vi "3_2_(1).vi"() -> ()   [LabVIEW 2010]
uses:
  Control 1.ctl
  Global 1.vi
panel:
  in  "Зчитати дані":bool
  out "Таблиця 1 - Вхідні дані":string[][](table)
  out "Таблиця 2 - Сортування":string[][](table)
  in  "4":bool
  in  "3":bool
  in  "2":bool
  in  "1":bool
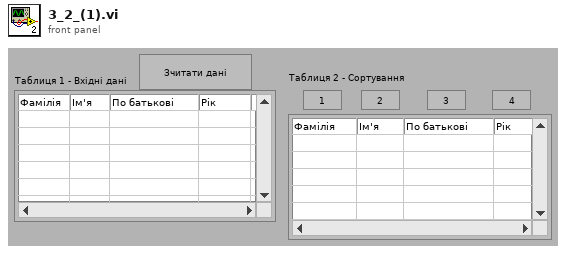
[diagram p1: front panel]
types:
  T1 = typedef "Control 1.ctl" = enum16{"Зчитати", "Стоп", "1", "2", "3", "4"}
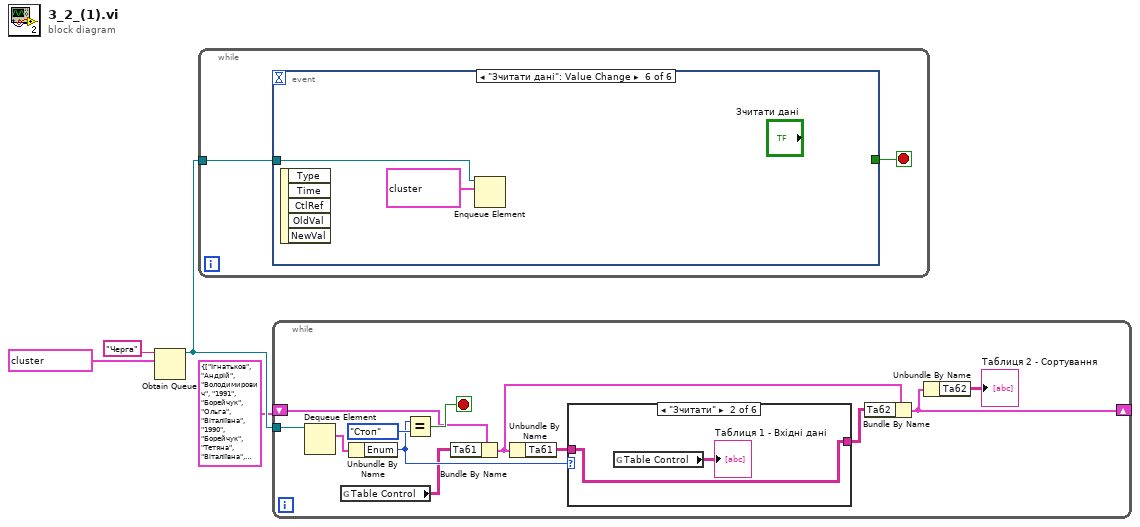
[diagram p0: block diagram]
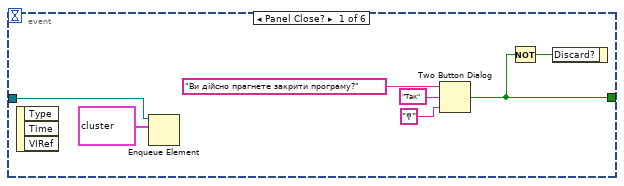
[diagram p2: hidden frame]
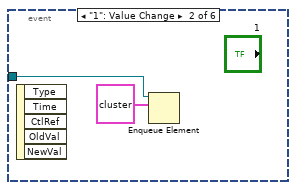
[diagram p3: hidden frame]
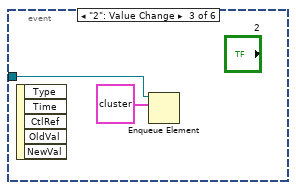
[diagram p4: hidden frame]
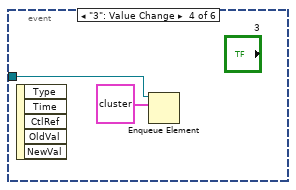
[diagram p5: hidden frame]
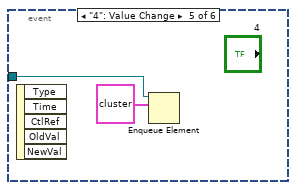
[diagram p6: hidden frame]
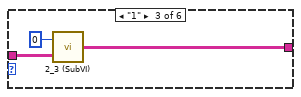
[diagram p8: hidden frame]
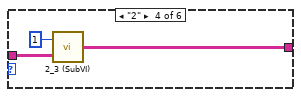
[diagram p9: hidden frame]
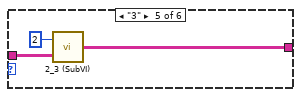
[diagram p10: hidden frame]
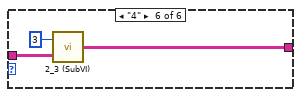
[diagram p11: hidden frame]
diagram:
  n1 = Obtain Queue(name (unnamed)="Черга", element data type=cluster{"variant":variant, "Enum":T1} {"variant"=variant, "Enum"=enum."Стоп"}) -> (queue out=w2:refnum<queue>)  [unwired: 3 in, 2 out]
  n2 = while {
    tunnel: w2 -> [w5]
    stop <- w6 stop-if-true
    n3 = event shown="[5] \"Зчитати дані\": Value Change" {
      selector: _ -> [_ _ _ _ _ _]
      dyn-events: _ -> [_ _ _ _ _ _]
      timeout: _ -> [_ _ _ _ _ _]
      tunnel: [w9 _ _ _ _ _] -> w6
      tunnel: w5 -> [w8 w14 w16 w18 w20 w22]
      event Panel Close? {
        n4 = event-data() -> ()  [unwired: 1 in, 3 out]
        n5 = Enqueue Element(queue=w8, element=cluster{"variant":variant, "Enum":T1} {"variant"=variant, "Enum"=enum."Стоп"}) -> ()  [unwired: 2 in, 3 out]
        n6 = Two Button Dialog(message="Ви дійсно прагнете закрити програму?", 1:"ͳ" ("F button name (\"Cancel\")"), 2:"Так" ("T button name (\"OK\")")) -> (T button?=w9:bool)
        n7 = Not(x=w9) -> (.not. x?=w10:bool)
        n8 = event-data("Discard?"=w10) -> ()  [unwired: 1 in, 1 out]
      }
      event "1": Value Change {
        n9 = event-data() -> ()  [unwired: 1 in, 5 out]
        n10 = Enqueue Element(queue=w14, element=cluster{"variant":variant, "Enum":T1} {"variant"=variant, "Enum"=enum."1"}) -> ()  [unwired: 2 in, 3 out]
      }
      event "2": Value Change {
        n11 = event-data() -> ()  [unwired: 1 in, 5 out]
        n12 = Enqueue Element(queue=w16, element=cluster{"variant":variant, "Enum":T1} {"variant"=variant, "Enum"=enum."2"}) -> ()  [unwired: 2 in, 3 out]
      }
      event "3": Value Change {
        n13 = event-data() -> ()  [unwired: 1 in, 5 out]
        n14 = Enqueue Element(queue=w18, element=cluster{"variant":variant, "Enum":T1} {"variant"=variant, "Enum"=enum."3"}) -> ()  [unwired: 2 in, 3 out]
      }
      event "4": Value Change {
        n15 = event-data() -> ()  [unwired: 1 in, 5 out]
        n16 = Enqueue Element(queue=w20, element=cluster{"variant":variant, "Enum":T1} {"variant"=variant, "Enum"=enum."4"}) -> ()  [unwired: 2 in, 3 out]
      }
      event "Зчитати дані": Value Change {
        n17 = event-data() -> ()  [unwired: 1 in, 5 out]
        n18 = Enqueue Element(queue=w22, element=cluster{"variant":variant, "Enum":T1} {"variant"=variant, "Enum"=enum."Зчитати"}) -> ()  [unwired: 2 in, 3 out]
      }
    }
  }
  n19 = while {
    tunnel: w2 -> [w35]
    shift-right: [w29] -> _
    shift-left: cluster{"Таб1":string[][], "Таб2":string[][]} {"Таб1"=[["Ігнатьков", "Андрій", "Володимирович", "1991"], ["Борейчук", "Ольга", "Віталіївна", "1990"], ["Борейчук", "Тетяна", "Віталіївна", "1990"], ["Котлубаєв", "Максим", "Євгенович", "1991"], ["Котлуьаєв", "Віталій", "Євгенович", "1989"]], "Таб2"=[["Ігнатьков", "Андрій", "Володимирович", "1991"], ["Борейчук", "Ольга", "Віталіївна", "1990"], ["Борейчук", "Тетяна", "Віталіївна", "1990"], ["Котлубаєв", "Максим", "Євгенович", "1991"], ["Котлуьаєв", "Віталій", "Євгенович", "1989"]]} -> [w25]
    stop <- w32 stop-if-true
    n20 = Dequeue Element(queue=w35) -> (element=w34:cluster{"variant":variant, "Enum":T1})  [unwired: 2 in, 3 out]
    n21 = global read "Global 1.vi" "Table Control"() -> (w26:string[][])
    n22 = Unbundle By Name(w34) -> ("Enum"=w31:T1)
    n23 = Equal?(x=w31, y=Control_1."Стоп" ("Enum")) -> (x = y?=w32:bool)
    n24 = Bundle By Name(cluster=w25, "Таб1"=w26) -> (w24:cluster{"Таб1":string[][], "Таб2":string[][]})
    n25 = Unbundle By Name(w24) -> ("Таб1"=w30:string[][])
    n26 = case shown="\"Зчитати\"" w31 {
      tunnel: w30 -> [w36 w37 w41 w42 w45 w49]
      tunnel: [w36 w37 w39 w44 w47 w48] -> w27
      frame "Стоп", Default {
      }
      frame "Зчитати" {
        n27 = global read "Global 1.vi" "Table Control"() -> (→"Таблиця 1 - Вхідні дані":string[][])
      }
      frame "1" {
        n28 = call "2_3 (SubVI).vi"("Таблиця 1 - Вхідні дані"=w41, "Сортувати стовпчик"=0) -> ("Таблиця 2 - Результат"=w39:string[][])
      }
      frame "2" {
        n29 = call "2_3 (SubVI).vi"("Таблиця 1 - Вхідні дані"=w42, "Сортувати стовпчик"=1) -> ("Таблиця 2 - Результат"=w44:string[][])
      }
      frame "3" {
        n30 = call "2_3 (SubVI).vi"("Таблиця 1 - Вхідні дані"=w45, "Сортувати стовпчик"=2) -> ("Таблиця 2 - Результат"=w47:string[][])
      }
      frame "4" {
        n31 = call "2_3 (SubVI).vi"("Таблиця 1 - Вхідні дані"=w49, "Сортувати стовпчик"=3) -> ("Таблиця 2 - Результат"=w48:string[][])
      }
    }
    n32 = Bundle By Name(cluster=w24, "Таб2"=w27) -> (w29:cluster{"Таб1":string[][], "Таб2":string[][]})
    n33 = Unbundle By Name(w29) -> ("Таб2"=→"Таблиця 2 - Сортування":string[][])
  }
